vi "Calibration.vi"() -> ()   [LabVIEW 2020, in "Setting Lib.lvlib"]
uses:
  Setting Lib.lvlib
  Database Lib.lvlib
panel:
  out "Height Ratio":dbl format="%.4f"
  out "Width Ratio":dbl format="%.4f"
  out "Height (Pixel)":i64
  in  "Real Height":i64
  out "Width (Pixel)":i64
  in  "Real Width":i64
  in  "Close":bool
  # "Calibration"
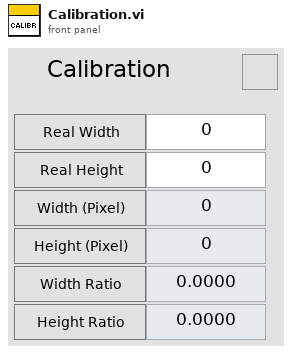
[diagram p1: front panel]
types:
  T1 = cluster{"Real Width":i64, "Real Height":i64, dbl, dbl}
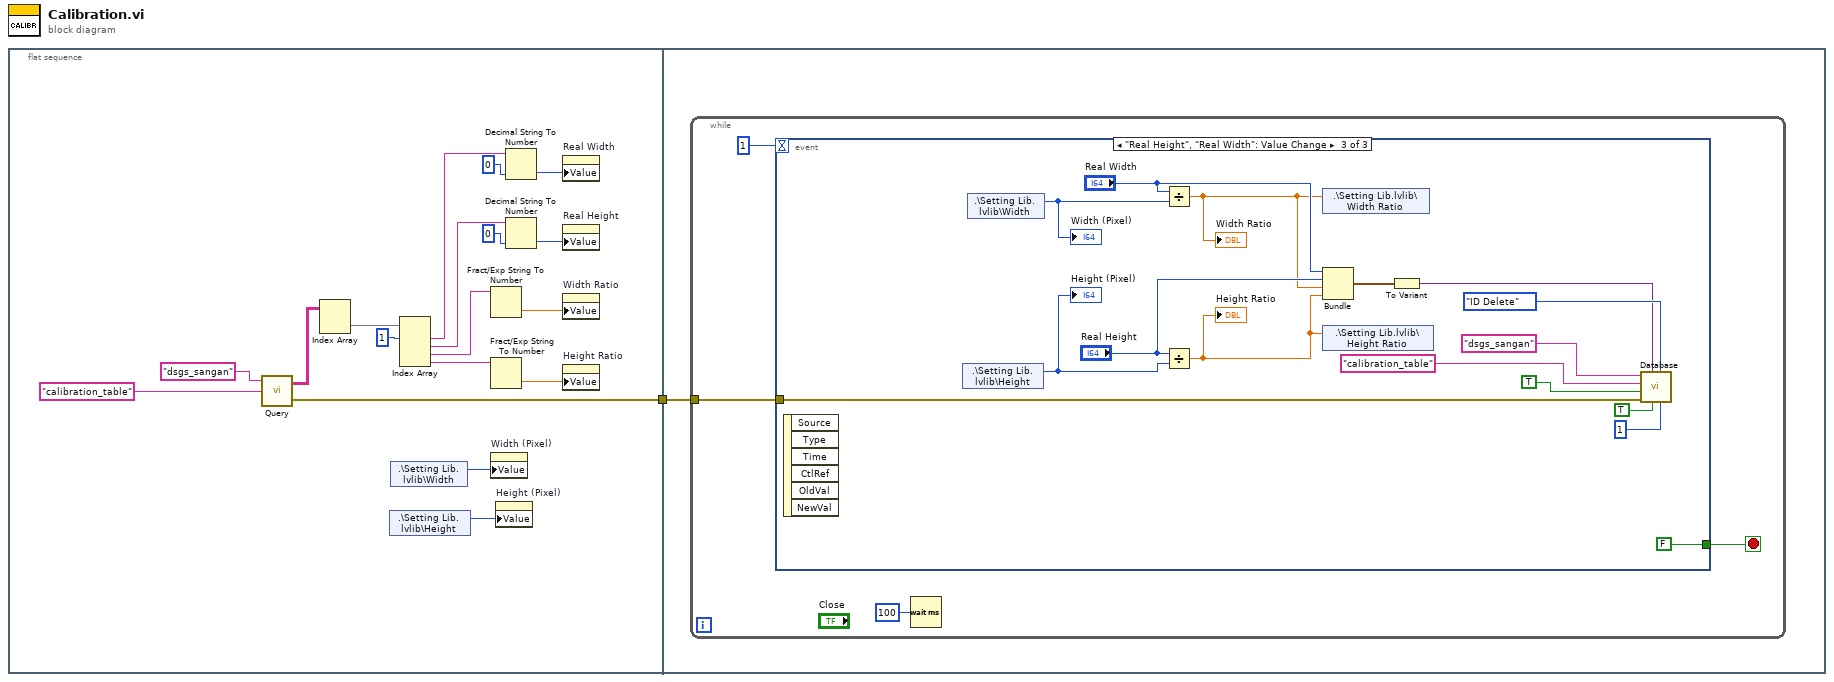
[diagram p0: block diagram]
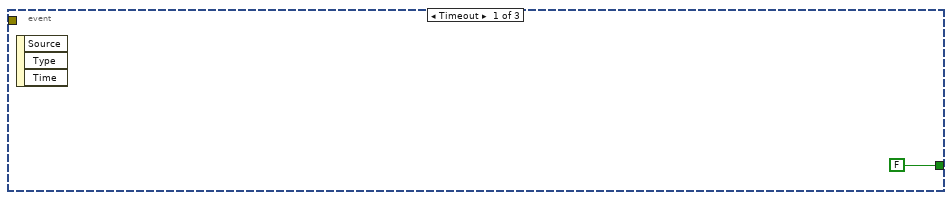
[diagram p2: hidden frame]
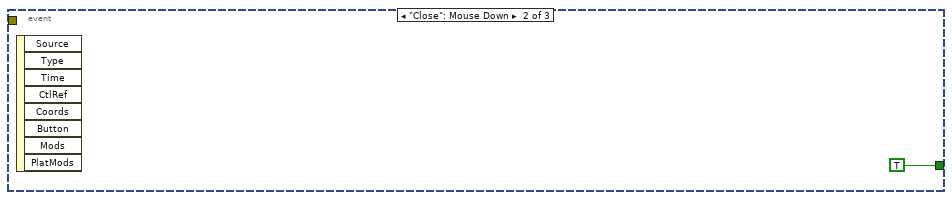
[diagram p3: hidden frame]
diagram:
  n1 = flat-sequence {
    tunnel: [w4] -> w1
    tunnel: w1 -> [w20]
    frame #0 {
      n2 = call "Query.vi"("Table Name"="calibration_table", "Connection Name"="dsgs_sangan") -> ("Error out"=w4:errorcluster, "data"=w10:string[][])  [unwired: 2 in]
      n3 = Index Array(array=w10) -> (element=w11:string[])  [unwired: 2 in]
      n4 = shared-variable ".\\Setting Lib.lvlib\\Height"() -> (w2:i64)  [unwired: 1 in, 1 out]
      n5 = shared-variable ".\\Setting Lib.lvlib\\Width"() -> (w3:i64)  [unwired: 1 in, 1 out]
      n6 = Index Array(array=w11, index #1=1 ("index")) -> (element #1=w12:string, element #2=w13:string, element #3=w16:string, element #4=w17:string)  [unwired: 3 in]
      n7 = Fract/Exp String To Number(string=w16) -> (number=w18:dbl)  [unwired: 3 in, 1 out]
      n8 = Fract/Exp String To Number(string=w17) -> (number=w19:dbl)  [unwired: 3 in, 1 out]
      n9 = property on="Width (Pixel)" class="DigNum (strict)"("Value"=w3) -> ()  [unwired: 2 in, 2 out]
      n10 = property on="Height (Pixel)" class="DigNum (strict)"("Value"=w2) -> ()  [unwired: 2 in, 2 out]
      n11 = Decimal String To Number(string=w12, default (0L)=i64 0 ("default (0 I32)")) -> (number=w14:i64)  [unwired: 1 in, 1 out]
      n12 = Decimal String To Number(string=w13, default (0L)=i64 0 ("default (0 I32)")) -> (number=w15:i64)  [unwired: 1 in, 1 out]
      n13 = property on="Real Width" class="DigNum (strict)"("Value"=w14) -> ()  [unwired: 2 in, 2 out]
      n14 = property on="Real Height" class="DigNum (strict)"("Value"=w15) -> ()  [unwired: 2 in, 2 out]
      n15 = property on="Width Ratio" class="DigNum (strict)"("Value"=w18) -> ()  [unwired: 2 in, 2 out]
      n16 = property on="Height Ratio" class="DigNum (strict)"("Value"=w19) -> ()  [unwired: 2 in, 2 out]
    }
    frame #1 {
      n17 = while {
        tunnel: w20 -> [w21]
        stop <- w22 stop-if-true
        n18 = event shown="[2] \"Real Height\", \"Real Width\": Value Change" {
          selector: _ -> [_ _ _]
          dyn-events: _ -> [_ _ _]
          timeout: 1 -> [_ _ _]
          tunnel: [FALSE TRUE FALSE] -> w22
          tunnel: w21 -> [_ _ w37]
          event Timeout {
            n19 = event-data() -> ()  [unwired: 1 in, 3 out]
          }
          event "Close": Mouse Down {
            n20 = event-data() -> ()  [unwired: 1 in, 8 out]
          }
          event "Real Height", "Real Width": Value Change {
            n21 = event-data() -> ()  [unwired: 1 in, 6 out]
            n22 = shared-variable ".\\Setting Lib.lvlib\\Height"() -> (w40:i64)  [unwired: 1 in, 1 out]
            "Height (Pixel)" <- w40
            n23 = shared-variable ".\\Setting Lib.lvlib\\Width"() -> (w41:i64)  [unwired: 1 in, 1 out]
            "Width (Pixel)" <- w41
            n24 = Divide(x="Real Width", y=w41) -> (x/y=w28:dbl)
            "Width Ratio" <- w28
            n25 = Divide(x="Real Height", y=w40) -> (x/y=w27:dbl)
            "Height Ratio" <- w27
            n26 = shared-variable ".\\Setting Lib.lvlib\\Width Ratio"(w28) -> ()  [unwired: 1 in, 1 out]
            n27 = Bundle("Real Width"="Real Width", "Real Height"="Real Height", w28, w27) -> (w30:T1)  [unwired: 1 in]
            n28 = shared-variable ".\\Setting Lib.lvlib\\Height Ratio"(w27) -> ()  [unwired: 1 in, 1 out]
            n29 = To Variant(anything=w30) -> (Variant=w29:variant)
            n30 = call "Database.vi"("Maximum Row"=1, "Enum"=enum16{"ID Delete", "Time Delete"}."ID Delete", "Delete row?"=TRUE, "Data"=w29, "Error in"=w37, "Auto Increment ID?"=TRUE, "Table"="calibration_table", "Connection"="dsgs_sangan") -> ()  [unwired: 3 in, 1 out]
          }
        }
        n31 = Wait (ms)(milliseconds to wait=u32 100) -> ()  [unwired: 1 out]
      }
    }
  }
